vi "Select UI Enable or Dis.vi"(6 "Disabled":T1(ring), 8 "error in (no error)":errorcluster, 10 "UI":string[](array[string]), 11 "Map In":map{string, refnum<vi>}(c390)) -> (0 "error out":errorcluster)   [LabVIEW 2020]
panel:
  out "Array":refnum<vi>[](array[refnum])
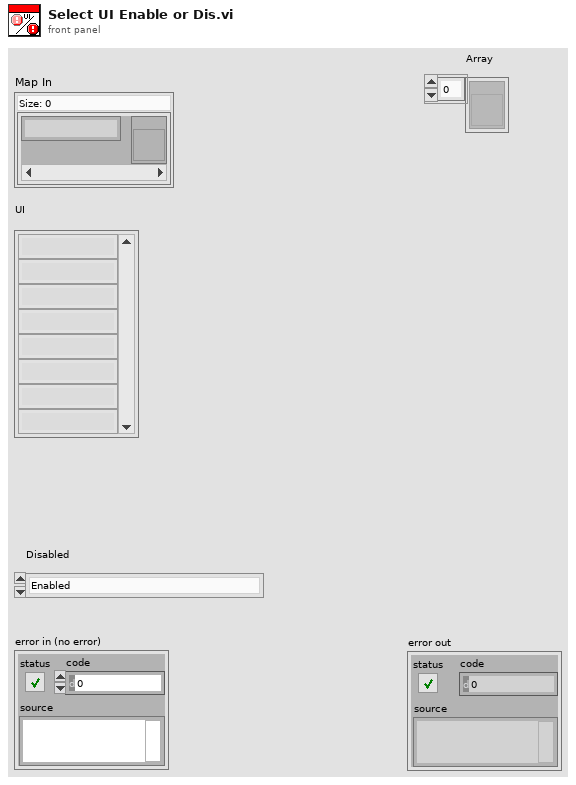
[diagram p1: front panel]
types:
  T1 = enum8{"Enabled", "Disabled", "Disabled and Grayed Out"}
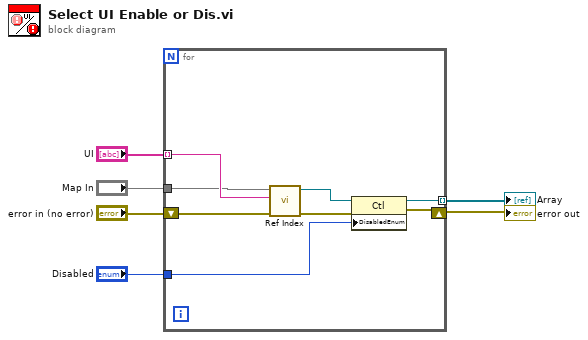
[diagram p0: block diagram]
diagram:
  n1 = for {
    shift-right: [w14] -> w5
    shift-left: "error in (no error)" -> [w13]
    tunnel: "UI" -> [w11] mode=indexing
    tunnel: "Map In" -> [w10]
    tunnel: [w8] -> w2 mode=indexing
    tunnel: "Disabled" -> [w7]
    n2 = call "Ref Index.vi"("error in"=w13, "Label"=w11, "Map Out"=w10) -> ("error out"=w12:errorcluster, "value"=w9:refnum<vi>)  [unwired: 6 in, 1 out]
    n3 = property class="Ctl"(reference=w9, error in=w12, "DisabledEnum"=w7) -> (reference out=w8:refnum<vi>, error out=w14:errorcluster)
  }
  "error out" <- w5
  "Array" <- w2
